vi "Start.vi"(11 "IO":T1) -> (3 "bt_Node out":refnum<class "bt_Node.lvclass">)   [LabVIEW 2021, in "Car Wash Support.lvlib"]
uses:
  Car Wash Support.lvlib
  IO Refs.ctl
  <vilib>/TSA/Event Log/Event_TextLog/Event_TextLog.lvclass
  C:/Program Files (x86)/National Instruments/LabVIEW 2021/vi.lib/TSA/Event Log/abs_EventLog/abs_EventLog.lvclass
  <vilib>/TSA/Abstract Data Classes/Abs_Types/Boolean/Abs_Boolean.lvclass
  C:/Program Files (x86)/National Instruments/LabVIEW 2021/vi.lib/TSA/Abstract Data Classes/Abs_Types/Type/Abs_Type.lvclass
  <vilib>/TSA/Abstract Data Classes/Abs_Types/I32 Integer/Abs_I32 Integer.lvclass
  <vilib>/TSA/Abstract Data Classes/Abs_Types/Double Float/Abs_Double Float.lvclass
  Wash Indicators.ctl
  Wash Options.ctl
  Support/Nodes/abs_Node/bt_Node.lvclass
  Support/Nodes/Decorators/Repeater/Support/Finish On - Type.ctl
  Support/Nodes/Leaves/abs_Type Leaf/abs_Type Leaf.lvclass/abs_Type Leaf.ctl
  Support/Nodes/Leaves/abs_Type Leaf/Properties/Write Value Class.vi
  Support/Nodes/Leaves/Test Boolean/Test Abs_Boolean.lvclass
  C:/Users/timst/Documents/Repositories/LV_Behaviour_Tree/Source/Support/Nodes/abs_Node/bt_Node.lvclass
  C:/Users/timst/Documents/Repositories/LV_Behaviour_Tree/Source/Support/Nodes/Leaves/abs_Type Leaf/abs_Type Leaf.lvclass
  Support/Nodes/Leaves/Log/bt_Log.lvclass
  <vilib>/TSA/Abstract Data Classes/Constants/Support/Str/Str.vi
  Support/Poly/Log/Log_StringClass.vi
  BT.lvlib
  Support/Nodes/Decorators/Repeater/bt_Repeater.lvclass
  <vilib>/TSA/Abstract Data Classes/Constants/Support/Str/Const_Str.lvclass
  C:/Program Files (x86)/National Instruments/LabVIEW 2021/vi.lib/TSA/Event Log/Event_TextLog/Event_TextLog.lvclass
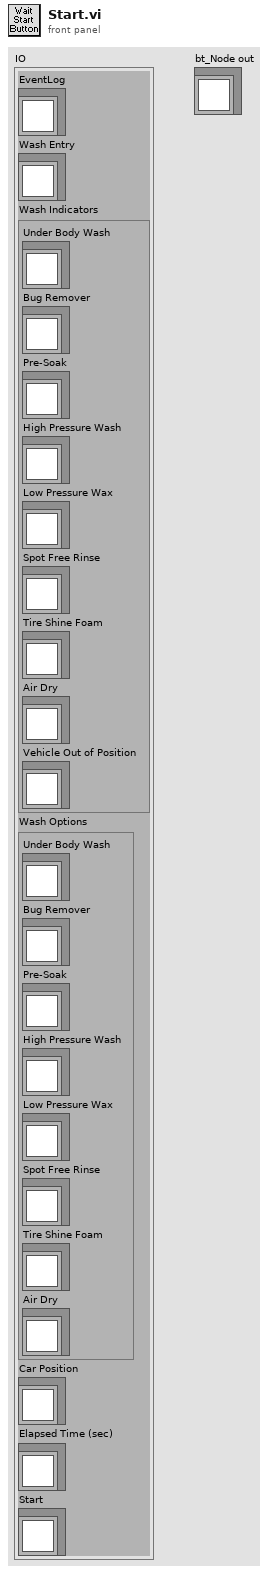
[diagram p1: front panel]
types:
  T1 = typedef "Car Wash Support.lvlib/IO Refs.ctl" = cluster{"EventLog":refnum<class "Event_TextLog.lvclass">, "Wash Entry":refnum<class "Abs_Boolean.lvclass">, "Wash Indicators":T2, "Wash Options":T3, "Car Position":refnum<class "Abs_I32 Integer.lvclass">, "Elapsed Time (sec)":refnum<class "Abs_Double Float.lvclass">, "Start":refnum<class "Abs_Boolean.lvclass">}
  T2 = typedef "Car Wash Support.lvlib/Wash Indicators.ctl" = cluster{"Under Body Wash":refnum<class "Abs_Boolean.lvclass">, "Bug Remover":refnum<class "Abs_Boolean.lvclass">, "Pre-Soak":refnum<class "Abs_Boolean.lvclass">, "High Pressure Wash":refnum<class "Abs_Boolean.lvclass">, "Low Pressure Wax":refnum<class "Abs_Boolean.lvclass">, "Spot Free Rinse":refnum<class "Abs_Boolean.lvclass">, "Tire Shine Foam":refnum<class "Abs_Boolean.lvclass">, "Air Dry":refnum<class "Abs_Boolean.lvclass">, "Vehicle Out of Position":refnum<class "Abs_Boolean.lvclass">}
  T3 = typedef "Car Wash Support.lvlib/Wash Options.ctl" = cluster{"Under Body Wash":refnum<class "Abs_Boolean.lvclass">, "Bug Remover":refnum<class "Abs_Boolean.lvclass">, "Pre-Soak":refnum<class "Abs_Boolean.lvclass">, "High Pressure Wash":refnum<class "Abs_Boolean.lvclass">, "Low Pressure Wax":refnum<class "Abs_Boolean.lvclass">, "Spot Free Rinse":refnum<class "Abs_Boolean.lvclass">, "Tire Shine Foam":refnum<class "Abs_Boolean.lvclass">, "Air Dry":refnum<class "Abs_Boolean.lvclass">}
  T4 = typedef "BT.lvlib/bt_Repeater.lvclass/Finish On - Type.ctl" = enum16{"Success", "Failure", "Never"}
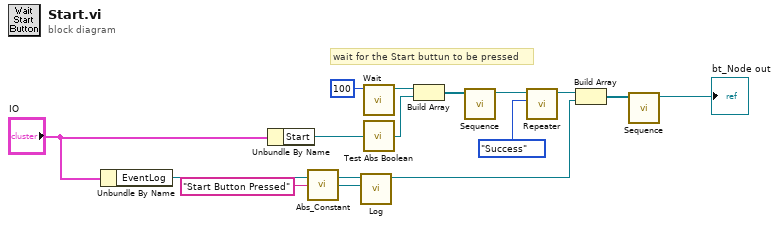
[diagram p0: block diagram]
diagram:
  # "wait for the Start buttun to be pressed"
  n1 = Unbundle By Name("IO") -> ("EventLog"=w14:refnum<class "Event_TextLog.lvclass">)
  n2 = Unbundle By Name("IO") -> ("Start"=w5:refnum<class "Abs_Boolean.lvclass">)
  n3 = call-poly <vilib>:"Abs_Constant.vi"("String"="Start Button Pressed") -> ("Abs_String.lvclass"=w12:refnum<class "Abs_String.lvclass">)  [unwired: 4 in]
  n4 = call-poly "Log.vi"("Message"=w12, "EventLog"=w14) -> ("node out"=w2:refnum<class "bt_Log.lvclass">)  [unwired: 9 in]
  n5 = call "Wait.vi"("Time (ms)"=u32 100) -> ("Node Out"=w10:refnum<class "bt_Node.lvclass">)  [unwired: 10 in]
  n6 = call "Test Abs Boolean.vi"("Abs_Boolean.lvclass"=w5) -> ("abs_Node"=w9:refnum<class "bt_Node.lvclass">)  [unwired: 4 in]
  n7 = Build Array(w10, w9) -> (w8:refnum<class "bt_Node.lvclass">[])
  n8 = call "Sequence.vi"("Nodes"=w8) -> ("Node"=w6:refnum<class "bt_Node.lvclass">)  [unwired: 10 in]
  n9 = call "Repeater.vi"("Finish On"=Finish_On_-_Type."Success", "Node In"=w6) -> ("Node Out"=w4:refnum<class "bt_Node.lvclass">)  [unwired: 9 in]
  n10 = Build Array(w4, w2) -> (w3:refnum<class "bt_Node.lvclass">[])
  n11 = call "Sequence.vi"("Nodes"=w3) -> ("Node"=→"bt_Node out":refnum<class "bt_Node.lvclass">)  [unwired: 10 in]
